vi "Mutate Log File Directory.vi"(8 "error in (no error)":errorcluster, 11 "Device Ref in":T1 format="%.0x") -> (0 "error out":errorcluster, 3 "Device Ref out":T1 format="%.0x")   [LabVIEW 2027, in "Embedded Data Logger System Explorer.lvlib"]
uses:
  Embedded Data Logger System Explorer.lvlib
  <vilib>/NI VeriStand/Custom Device API/Custom Device Item Ref.ctl
  <vilib>/NI VeriStand/Custom Device Tools/Custom Device Utility Library/NI VeriStand - Search for All Items by GUID.vi
  <vilib>/NI VeriStand/Custom Device API/Get Item Property (Path).vi
  <vilib>/NI VeriStand/Custom Device API/Set Item Property (String Array).vi
  <vilib>/NI VeriStand/Custom Device Tools/Custom Device Utility Library/Custom Device Utility Library.lvlib
  <vilib>/NI VeriStand/Custom Device API/Custom Device API.lvlib
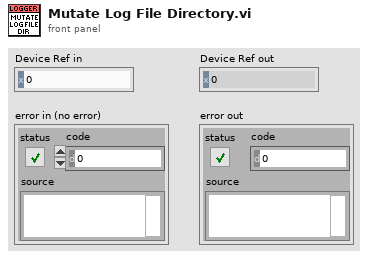
[diagram p1: front panel]
types:
  T1 = typedef "Custom Device API.lvlib/Custom Device Item Ref.ctl" = u64
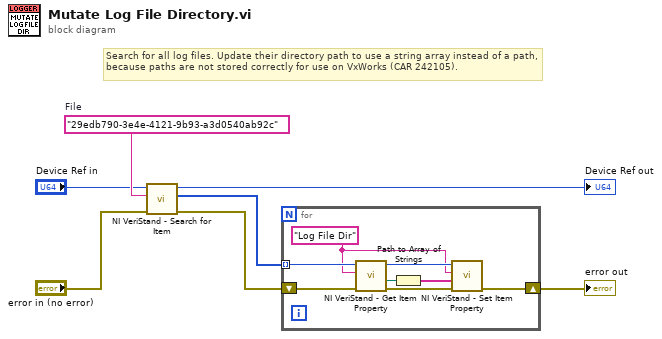
[diagram p0: block diagram]
diagram:
  w7 = "29edb790-3e4e-4121-9b93-a3d0540ab92c"  # File
  # "Search for all log files. Update their directory path to use a string array instead of a path, because paths are not stored correctly for use on VxWorks (CAR 242105)."
  n1 = call-poly <vilib>:"NI VeriStand - Search for Item.vi"("error in"="error in (no error)", "Item GUID"=w7, "Section Ref in"="Device Ref in") -> ("error out"=w4:errorcluster, "Item Refs"=w5:T1[], "Section Ref out"=→"Device Ref out":T1)  [unwired: 1 in, 5 out]
  n2 = for {
    shift-right: [w8] -> w6
    shift-left: w4 -> [w15]
    tunnel: w5 -> [w14] mode=indexing
    w9 = "Log File Dir" ("Property Name")
    n3 = call-poly <vilib>:"NI VeriStand - Get Item Property.vi"("error in (no error)"=w15, "Property Name"=w9, "Item Ref in"=w14) -> ("error out"=w13:errorcluster, "Value"=w11:path, "Item Ref out"=w12:T1)  [unwired: 5 in, 1 out]
    n4 = Path to Array of Strings(0:w11) -> (2:w10:string[])  [unwired: 1 out]
    n5 = call-poly <vilib>:"NI VeriStand - Set Item Property.vi"("error in (no error)"=w13, "Value"=w10, "Property Name"=w9, "Item Ref in"=w12) -> ("error out"=w8:errorcluster)  [unwired: 5 in, 2 out]
  }
  "error out" <- w6
